vi "SubVI_SingleRead.vi"(7 "error in":errorcluster, 10 "String":string) -> (0 "error out":errorcluster, 2 "RData":variant, 3 "Read status?":bool)   [LabVIEW 2023, in "ADS_Library.lvlib"]
doc: "Single TwinCAT value read, this VI creates a connection to a TwinCAT parameter.\nThe parameter is read once and cast to LV types, the handle is then released and data \npassed out in an variant."
uses:
  ADS_Library.lvlib
  <userlib>/Beckhoff-LabVIEW-Interface/_DependsOn/Base/Read/Read Sync.vi
  <userlib>/Beckhoff-LabVIEW-Interface/_DependsOn/Base/TypeResolver/Get TypeResolver.vi
panel:
  out "RDataArray":variant[](array[variant])
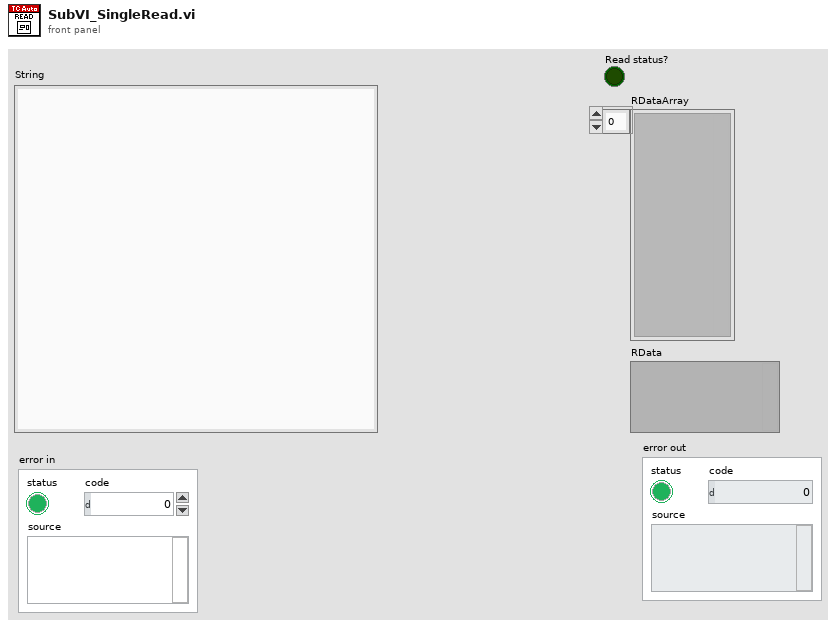
[diagram p1: front panel]
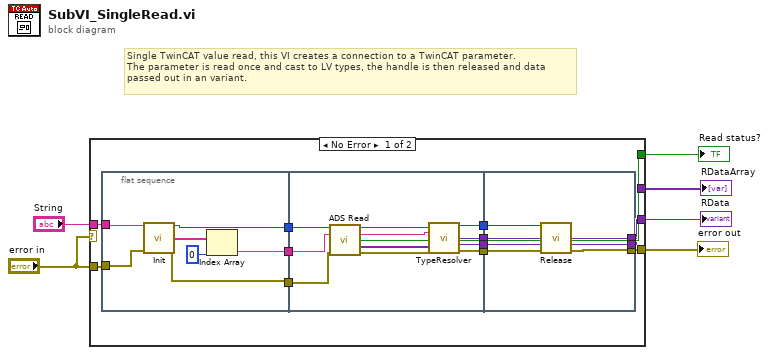
[diagram p0: block diagram]
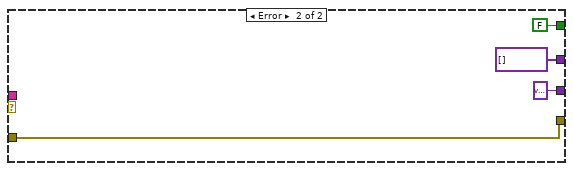
[diagram p2: hidden frame]
diagram:
  # "Single TwinCAT value read, this VI creates a connection to a TwinCAT parameter.\nThe parameter is read once and cast to LV types, the handle is then released and data \npassed out in an variant."
  n1 = case shown="No Error" "error in" {
    tunnel: "String" -> [w12 _]
    tunnel: "error in" -> [w11 w49]
    tunnel: [w10 w49] -> w5
    tunnel: [w9 FALSE ("Read status?")] -> w4
    tunnel: [w8 variant[] [] ("RDataArray")] -> w3
    tunnel: [w7 variant ("RData")] -> w2
    frame No Error {
      n2 = flat-sequence {
        tunnel: w12 -> [w27]
        tunnel: w11 -> [w26]
        tunnel: [w23] -> w20
        tunnel: [w22] -> w19
        tunnel: [w21] -> w18
        tunnel: [w37] -> w17
        tunnel: [w36] -> w16
        tunnel: w20 -> [w35]
        tunnel: w19 -> [w34]
        tunnel: w18 -> [w33]
        tunnel: [w31] -> w15
        tunnel: [w29] -> w14
        tunnel: [w28] -> w13
        tunnel: [w45] -> w10
        tunnel: w17 -> [w44]
        tunnel: w16 -> [w43]
        tunnel: [w42] -> w9
        tunnel: w15 -> [w42]
        tunnel: [w41] -> w8
        tunnel: w14 -> [w41]
        tunnel: [w40] -> w7
        tunnel: w13 -> [w40]
        frame #0 {
          n3 = call <userlib>:"Init.vi"("XMLDescription"=w27, "error in (no error)"=w26) -> ("Handle"=w21:u32, "ReadGrpSymbols"=w25:string[], "error out"=w23:errorcluster)  [unwired: 9 in, 2 out]
          n4 = Index Array(array=w25, index=0) -> (element=w22:string)
        }
        frame #1 {
          n5 = call-poly <userlib>:"ADS Read.vi"("Handle"=w33, "SymbolName"=w34, "error in (no error)"=w35) -> ("Handle"=w39:u32, "SymbolName"=w32:string, "Read status?"=w31:bool, "Ads Read Data"=w30:variant[], "error out"=w38:errorcluster)  [unwired: 8 in]
          n6 = call-poly <userlib>:"TypeResolver.vi"("Handle"=w39, "SymbolName"=w32, "ADSRData"=w30, "error in"=w38) -> ("Handle"=w37:u32, "RDataArray"=w29:variant[], "RData"=w28:variant, "error out"=w36:errorcluster)  [unwired: 8 in]
        }
        frame #2 {
          n7 = call <userlib>:"Release.vi"("Handle"=w44, "error in (no error)"=w43) -> ("error out"=w45:errorcluster)  [unwired: 13 in]
        }
      }
    }
    frame Error {
    }
  }
  "Read status?" <- w4
  "RDataArray" <- w3
  "error out" <- w5
  "RData" <- w2
